vi "Sub_MotorR.vi"(1 "R":i32) -> (0 "문자열":string)   [LabVIEW 2013]
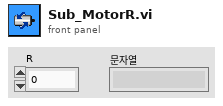
[diagram p1: front panel]
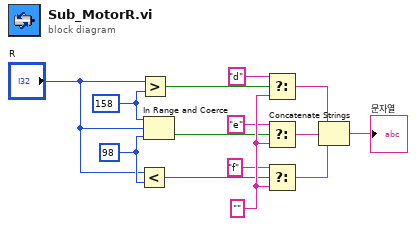
[diagram p0: block diagram]
diagram:
  w14 = ""
  w5 = 98
  w6 = 158
  n1 = Less?(x="R", y=w5) -> (x < y?=w4:bool)
  n2 = Greater?(x="R", y=w6) -> (0:w2:bool)
  n3 = In Range and Coerce(upper limit=w6, x="R", lower limit=w5) -> (In Range?=w3:bool)  [unwired: 1 out]
  n4 = Select(t="d", s=w2, f=w14) -> (s? t:f=w10:string)
  n5 = Select(t="e", s=w3, f=w14) -> (s? t:f=w11:string)
  n6 = Select(t="f", s=w4, f=w14) -> (s? t:f=w12:string)
  n7 = Concatenate Strings(w10, w11, w12) -> (→"문자열":string)
